vi "Manage Collision.vi"(11 "Collision in":refnum<class "Collision.lvclass">) -> (1 "Remove GB Components out":refnum<class "Game Board Component.lvclass">[](array[class]), 2 "Insert GB Components out":refnum<class "Game Board Component.lvclass">[](array[class]))   [LabVIEW 2024, in "Collision.lvclass"]
doc: "MIT Licence\nCopyright (c) 2024 David Grollier"
uses:
  Collision.lvclass
  Game Componants/Game Board Component/Game Board Component.lvclass
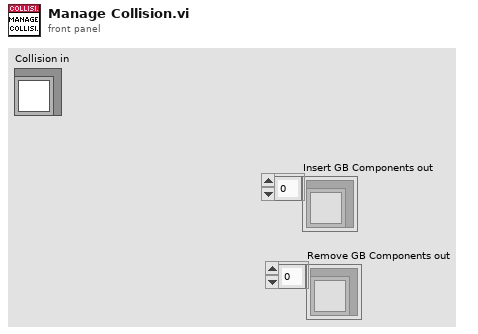
[diagram p1: front panel]
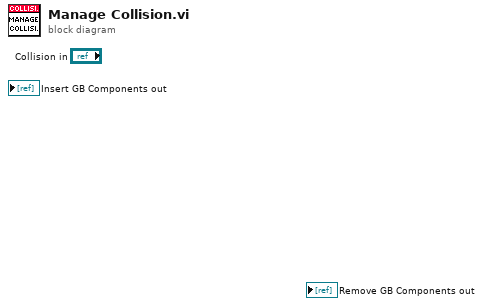
[diagram p0: block diagram]
diagram:
